vi "Write PropertyNewValue.vi"(8 "error in (no error)":errorcluster, 10 "PropertyNewValue":string, 11 "TektronixDPO in":refnum<class "TektronixDPO.lvclass">) -> (0 "error out":errorcluster, 3 "TektronixDPO out":refnum<class "TektronixDPO.lvclass">)   [LabVIEW 2013, in "TektronixDPO.lvclass"]
uses:
  TektronixDPO.lvclass
  TektronixDPO.lvclass/TektronixDPO.ctl
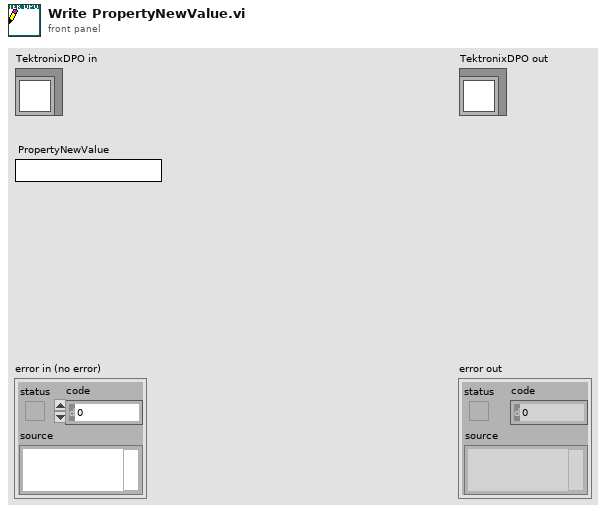
[diagram p1: front panel]
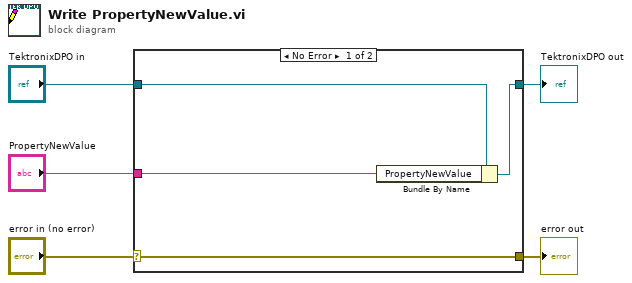
[diagram p0: block diagram]
diagram:
  n1 = case shown="No Error" "error in (no error)" {
    selector: "error in (no error)" -> [w9 w10]
    tunnel: [w9 w10] -> w4
    tunnel: [w7 w11] -> w2
    tunnel: "TektronixDPO in" -> [w8 w11]
    tunnel: "PropertyNewValue" -> [w6 _]
    frame No Error {
      n2 = Bundle By Name(cluster=w8, "PropertyNewValue"=w6) -> (w7:refnum<class "TektronixDPO.lvclass">)
    }
    frame Error {
    }
  }
  "error out" <- w4
  "TektronixDPO out" <- w2
